vi "VALEW_Sensors_Pressure_Redundant.vi"(0 "GEA2 Reference In":refnum<k24>, 1 "Lim_L_R_Pressure (inches)":dbl[](array[numeric])=[2.0, 7.0, 12.0, 17.0, 20.0], 3 "Lim_U_R_Pressure (inches)":dbl[](array[numeric])=[2.0, 7.0, 12.0, 17.0, 20.0], 5 "GEA Inputs":T1={"Source"=228, "Destination"=35} {"Destination" format="%.0x"; "Source" format="%.0x"}, 7 "DAQmx Physical Channel":tag="9263_1/ao0", 9 "Array of Voltages":dbl[](array[numeric])=[1.0, 2.0, 3.0, 4.0, 5.0], 10 "Standalone?":bool=TRUE, 11 "Error In":errorcluster, 12 "Lim_L_Pressure (inches of water)":dbl[](array[numeric])=[2.0, 7.0, 12.0, 17.0, 20.0], 14 "Lim_U_Pressure (inches of water)":dbl[](array[numeric])=[4.0, 8.0, 13.0, 18.0, 21.0]) -> (2 "Redundant PS (Inches )":dbl[](array[numeric]), 4 "GEA2 Reference Out":refnum<k24>, 6 "Pass/Fail?":bool, 8 "Report Text":string, 13 "Pressure (inches of water)":dbl[](array[numeric]), 15 "Error Out":errorcluster)   [LabVIEW 2016, in "TL27.lvlib"]
uses:
  Projects/TL27.lvlib
  C:/Automation/DLLs/PC Dot Net/GeaCommunication.dll
  Common/LabVIEW GEA2 Toolkit/LabVIEW_GEA2_Toolkit.lvlibp/type defs/Source_Destination.ctl
  Common/LabVIEW GEA2 Toolkit/LabVIEW_GEA2_Toolkit.lvlibp/type defs/ERD Read Data In.ctl
  Common/LabVIEW GEA2 Toolkit/LabVIEW_GEA2_Toolkit.lvlibp/type defs/Data Type.ctl
  <vilib>/DAQmx/write.llb/DAQmx Write (Analog DBL 1Chan 1Samp).vi
  <vilib>/DAQmx/create/channels.llb/DAQmx Create Channel (AO-Voltage-Basic).vi
  <vilib>/DAQmx/miscellaneous.llb/DAQmx Fill In Error Info.vi
  Common/LabVIEW GEA2 Toolkit/LabVIEW_GEA2_Toolkit.lvlibp
panel:
  out "Pressure ADC":dbl[](array[numeric])
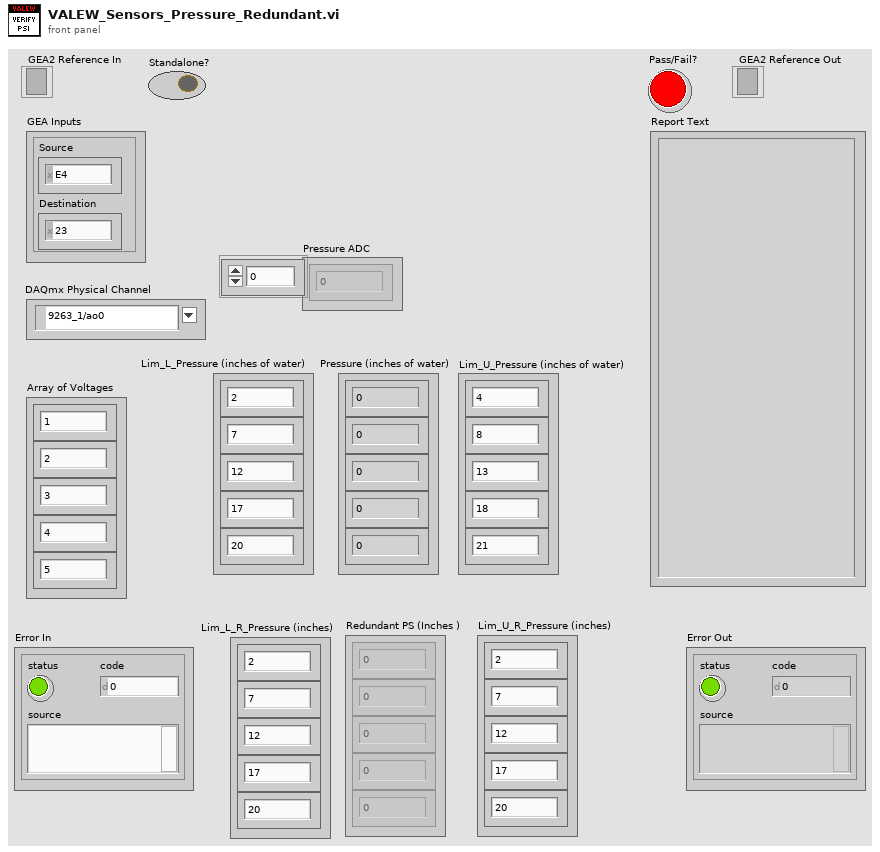
[diagram p1: front panel]
types:
  T1 = typedef "LabVIEW_GEA2_Toolkit.lvlibp/Source_Destination.ctl" = cluster{"Source":u8, "Destination":u8}
  T2 = typedef "LabVIEW_GEA2_Toolkit.lvlibp/ERD Read Data In.ctl" = cluster{"ERD Number":u16, "Data Type":T3}
  T3 = typedef "LabVIEW_GEA2_Toolkit.lvlibp/Data Type.ctl" = enum16{"string", "boolean", "uint8_t", "uint16_t", "uint32_t", "uint64_t", "int8_t", "int16_t", "int32_t", "int64_t"}
  T4 = typedef "LabVIEW_GEA2_Toolkit.lvlibp/ERD Read Data Out.ctl" = cluster{"ERD Number":u16, "Data":string}
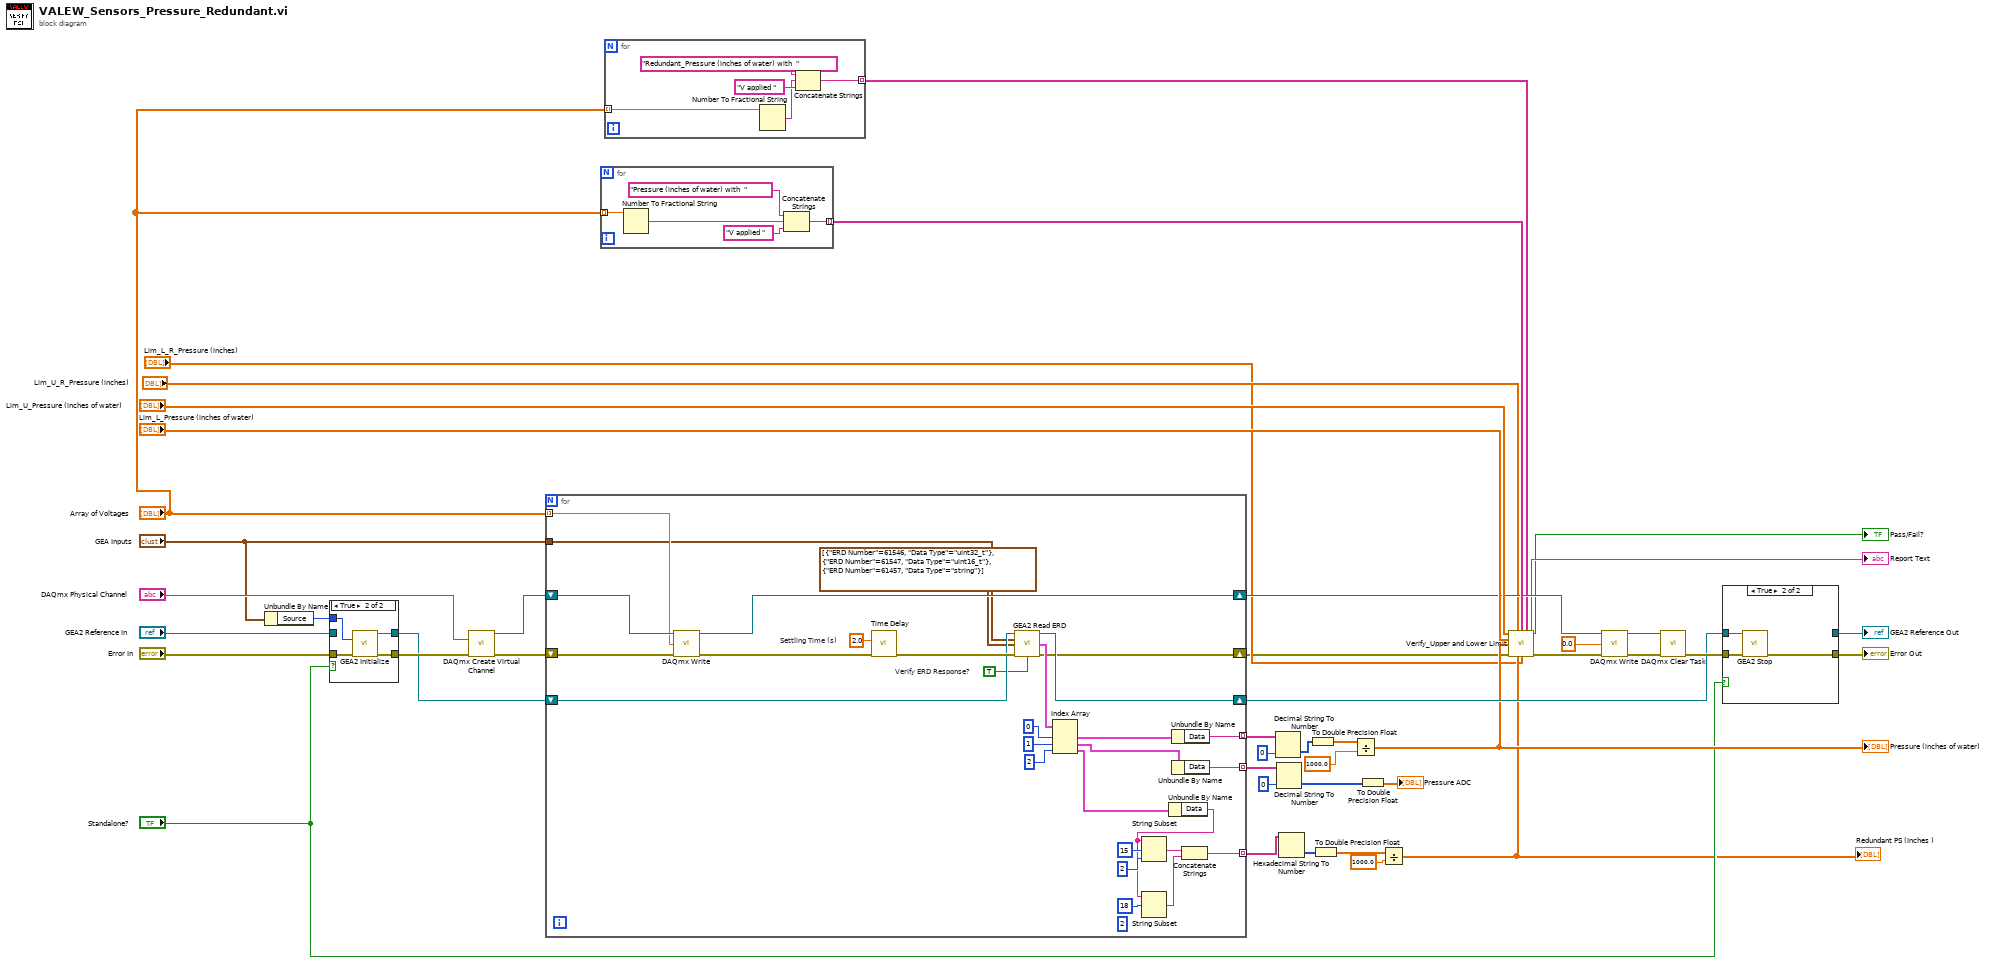
[diagram p0: block diagram]
diagram:
  n1 = Unbundle By Name("GEA Inputs") -> ("Source"=w33:u8)
  n2 = case shown="True" "Standalone?" {
    tunnel: "Error In" -> [w46 w50]
    tunnel: [w46 w49] -> w41
    tunnel: "GEA2 Reference In" -> [w45 _]
    tunnel: [w45 w48] -> w35
    tunnel: w33 -> [_ w47]
    frame False {
    }
    frame True {
      n3 = call "GEA2 Initialize.vi"("Source Address"=w47, "error in"=w50) -> ("GEA2 Reference Out"=w48:refnum<k24>, "error out"=w49:errorcluster)  [unwired: 11 in, 1 out]
    }
  }
  n4 = call-poly <vilib>:"DAQmx Create Virtual Channel.vi"("physical channels"="DAQmx Physical Channel", "error in"=w41) -> ("task out"=w38:refnum<k21>, "error out"=w40:errorcluster)  [unwired: 12 in]
  n5 = for {
    shift-right: [w61] -> w34
    shift-left: w35 -> [w73]
    shift-right: [w78] -> w15
    shift-left: w38 -> [w77]
    shift-right: [w60] -> w1
    shift-left: w40 -> [w79]
    tunnel: "GEA Inputs" -> [w66]
    tunnel: "Array of Voltages" -> [w72] mode=indexing
    tunnel: [w69] -> w31 mode=indexing
    tunnel: [w68] -> w28 mode=indexing
    tunnel: [w51] -> w10 mode=indexing
    (unwired) 2 ("length (rest)")
    w67 = TRUE  # Verify ERD Response?
    w76 = 2.0  # Settling Time (s)
    n6 = call-poly <vilib>:"DAQmx Write.vi"("task/channels in"=w77, "data"=w72, "error in"=w79) -> ("task out"=w78:refnum<k21>, "error out"=w74:errorcluster)  [unwired: 10 in, 1 out]
    n7 = call "Time Delay"("error in (no error)"=w74, "Delay Time (s)"=w76) -> ("error out"=w75:errorcluster)  [unwired: 9 in]
    n8 = call "GEA2 Read ERD.vi"("GEA2 Reference In"=w73, "GEA Inputs"=w66, "Read ERD List"=T2[] [{"ERD Number"=61546, "Data Type"=enum."uint32_t"}, {"ERD Number"=61547, "Data Type"=enum."uint16_t"}, {"ERD Number"=61457, "Data Type"=enum."string"}], "Error In"=w75, "Verify ERD Response?"=w67) -> ("GEA2 Reference Out"=w61:refnum<k24>, "ERD Data Out"=w71:T4[], "Error Out"=w60:errorcluster)  [unwired: 7 in, 1 out]
    n9 = Index Array(array=w71, index #1=0 ("index"), index #2=1 ("index"), index #3=2 ("index")) -> (element #1=w64:T4, element #2=w63:T4, element #3=w58:T4)
    n10 = Unbundle By Name(w58) -> ("Data"=w52:string)
    n11 = String Subset(string=w52, offset (0)=15, length (rest)=2 ("length (rest)")) -> (substring=w56:string)
    n12 = String Subset(string=w52, offset (0)=18) -> (substring=w57:string)  [unwired: 1 in]
    n13 = Unbundle By Name(w64) -> ("Data"=w68:string)
    n14 = Unbundle By Name(w63) -> ("Data"=w69:string)
    n15 = Concatenate Strings(w56, w57) -> (w51:string)
  }
  n16 = for {
    tunnel: "Array of Voltages" -> [w84] mode=indexing
    tunnel: [w80] -> w20 mode=indexing
    n17 = Number To Fractional String(number=w84) -> (F-format string=w81:string)  [unwired: 3 in]
    n18 = Concatenate Strings("Pressure (inches of water) with  ", w81, "V applied ") -> (w80:string)
  }
  n19 = for {
    tunnel: "Array of Voltages" -> [w89] mode=indexing
    tunnel: [w86] -> w8 mode=indexing
    n20 = Number To Fractional String(number=w89) -> (F-format string=w87:string)  [unwired: 3 in]
    n21 = Concatenate Strings("Redundant_Pressure (inches of water) with  ", w87, "V applied ") -> (w86:string)
  }
  n22 = Decimal String To Number(string=w28, default (0L)=u32 0 ("default (0 I32)")) -> (number=w24:u32[])  [unwired: 1 in, 1 out]
  n23 = Decimal String To Number(string=w31, default (0L)=u16 0 ("default (0 I32)")) -> (number=w27:u16[])  [unwired: 1 in, 1 out]
  n24 = Hexadecimal String To Number(string=w10) -> (number=w13:u32[])  [unwired: 2 in, 1 out]
  n25 = To Double Precision Float(number=w24) -> (double precision float=w25:dbl[])
  n26 = To Double Precision Float(number=w13) -> (double precision float=w12:dbl[])
  n27 = Divide(x=w25, y=1000.0) -> (x/y=w23:dbl[])
  "Pressure (inches of water)" <- w23
  n28 = To Double Precision Float(number=w27) -> (double precision float=→"Pressure ADC":dbl[])
  n29 = Divide(x=w12, y=1000.0) -> (x/y=w7:dbl[])
  "Redundant PS (Inches )" <- w7
  n30 = call "Verify_Upper and Lower Limit.vi"("Upper Limits"="Lim_U_Pressure (inches of water)", "R_Upper Limits"="Lim_U_R_Pressure (inches)", "Array of Names"=w20, "R_Array of Names"=w8, "Lower Limits"="Lim_L_Pressure (inches of water)", "Results"=w23, "Error In"=w1, "R_Results"=w7, "R_Lower Limits"="Lim_L_R_Pressure (inches)") -> ("Pass/Fail?"=→"Pass/Fail?":bool, "Report Text"=→"Report Text":string, "Error Out"=w18:errorcluster)  [unwired: 3 in, 1 out]
  n31 = call-poly <vilib>:"DAQmx Write.vi"("task/channels in"=w15, "data"=0.0, "error in"=w18) -> ("task out"=w16:refnum<k21>, "error out"=w17:errorcluster)  [unwired: 10 in, 1 out]
  n32 = call <vilib>:"DAQmx Clear Task.vi"("task in"=w16, "error in"=w17) -> ("error out"=w39:errorcluster)  [unwired: 13 in]
  n33 = case shown="True" "Standalone?" {
    tunnel: [w90 w94] -> w36
    tunnel: w34 -> [w91 w92]
    tunnel: [w91 _] -> w37
    tunnel: w39 -> [w90 w93]
    frame False {
    }
    frame True {
      n34 = call "GEA2 Stop.vi"("GEA2 Reference In"=w92, "Error In"=w93) -> ("Error Out"=w94:errorcluster)  [unwired: 13 in]
    }
  }
  "Error Out" <- w36
  "GEA2 Reference Out" <- w37
